vi "determine tempos.vi"(8 "error in (no error)":errorcluster, 11 "midi-file-events in":refnum<class "midi-file-events.lvclass">) -> (0 "error out":errorcluster, 2 "Track data by Track number":T1(c390), 3 "midi-file-events out":refnum<class "midi-file-events.lvclass">)   [LabVIEW 2020, in "midi-file-events.lvclass"]
uses:
  midi-file-events.lvclass
  midi-file-event.midi/midi-file-event.midi.lvclass
  C:/code/LabVIEW-MIDI/lv-src/midi-file-event/midi-file-event.lvclass
  midi-file-events.lvclass/midi-file-events.ctl
  midi-file-event/midi-file-event.lvclass/midi-file-event.ctl
  midi-file-event/Delta Tiime.get.vi
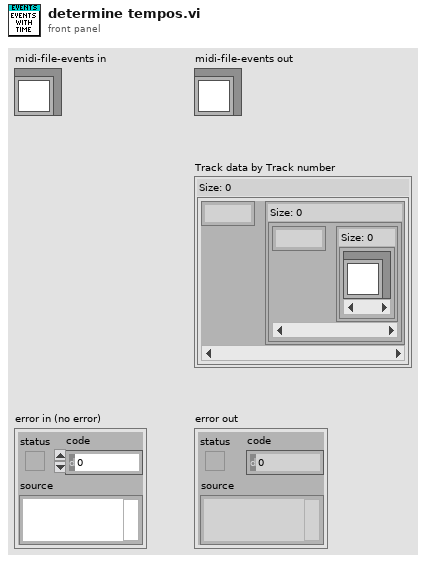
[diagram p1: front panel]
types:
  T1 = map{i32, map{dbl, set{refnum<class "midi-file-event.midi.lvclass">}}}
  T2 = map{dbl, set{refnum<class "midi-file-event.midi.lvclass">}}
  T3 = set{refnum<class "midi-file-event.midi.lvclass">}
  T4 = typedef "midi-file-events.lvclass/privatedata.ctl" = cluster{"ticks per quarter note (division)":i16, "Tempo Map":map{dbl, dbl}, "Track data by Track number":map{i32, map{dbl, set{refnum<class "midi-file-event.midi.lvclass">}}}}
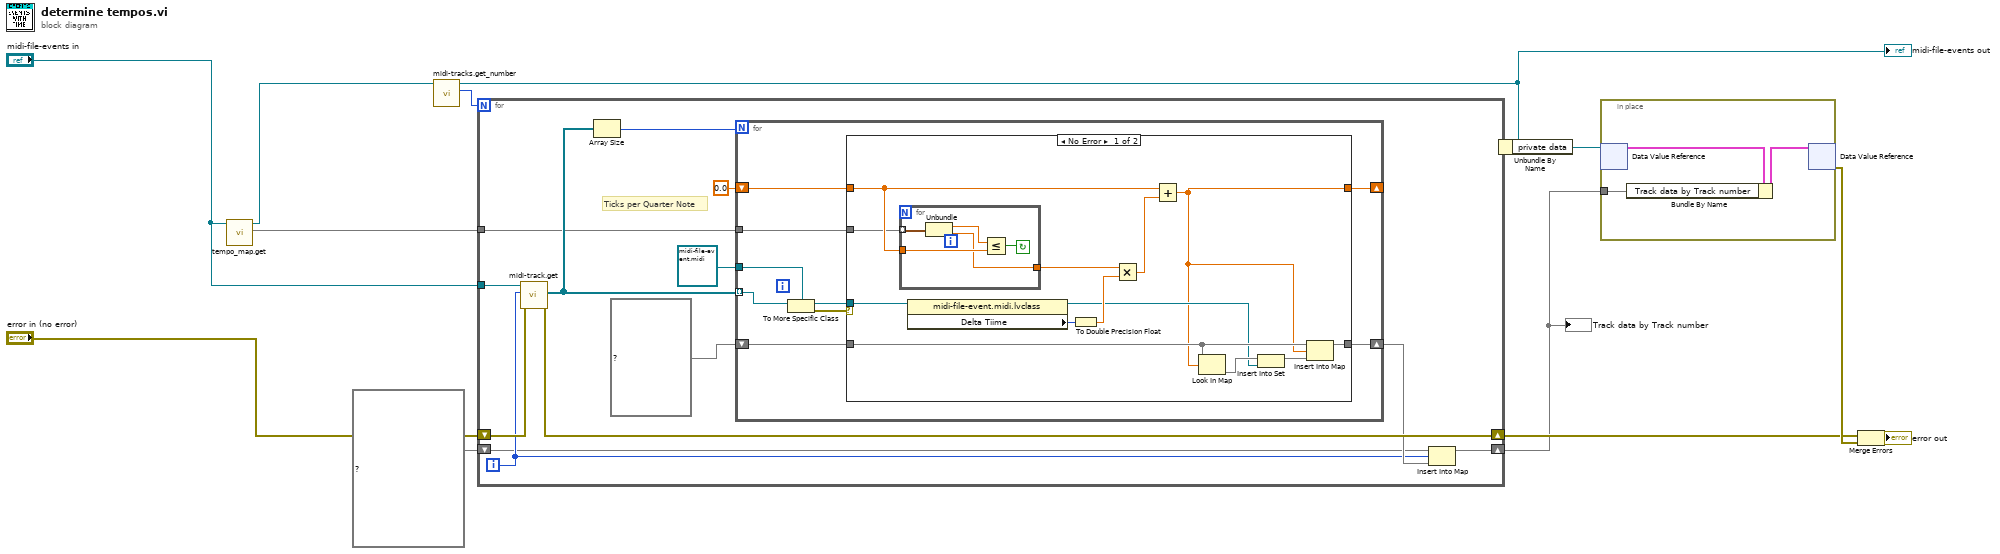
[diagram p0: block diagram]
diagram:
  n1 = call "tempo_map.get.vi"("midi-file-events in"="midi-file-events in") -> ("Tempo Map"=w1:map{dbl, dbl}, "midi-file-events out"=w8:refnum<class "midi-file-events.lvclass">)  [unwired: 8 in, 1 out]
  n2 = call "midi-tracks.get_number.vi"("midi-file-events in"=w8) -> ("Numer of Tracks"=w11:i32, "midi-file-events out"=w7:refnum<class "midi-file-events.lvclass">)  [unwired: 8 in, 1 out]
  "midi-file-events out" <- w7
  n3 = for {
    N: w11 -> [_]
    tunnel: "midi-file-events in" -> [w21]
    shift-right: [w25] -> w4
    shift-left: "error in (no error)" -> [w24]
    shift-right: [w17] -> w2
    shift-left: T1 {} ("Track data by Track number") -> [w18]
    tunnel: w1 -> [w13]
    i -> [w19]
    # "Ticks per Quarter Note"
    n4 = call "midi-track.get.vi"("error in (no error)"=w24, "Track Number"=w19, "midi-file-events in"=w21) -> ("error out"=w25:errorcluster, "file events"=w14:refnum<class "midi-file-event.lvclass">[])  [unwired: 6 in, 1 out]
    n5 = Array Size(array=w14) -> (size(s)=w23:i32)
    n6 = for {
      N: w23 -> [_]
      shift-right: [w33] -> _
      shift-left: 0.0 ("microseconds per quarter note") -> [w34]
      shift-right: [w31] -> w20
      shift-left: T2 {} ("midi event by timestamp") -> [w32]
      tunnel: refnum<class "midi-file-event.midi.lvclass"> refnum ("midi-file-event.midi.lvclass") -> [w30]
      tunnel: w14 -> [w28] mode=indexing
      tunnel: w13 -> [w26]
      n7 = To More Specific Class(target class=w30, reference=w28) -> (specific class reference=w27:refnum<class "midi-file-event.midi.lvclass">, error out=w29:errorcluster)  [unwired: 1 in]
      n8 = case shown="No Error" w29 {
        tunnel: w34 -> [w46 w54]
        tunnel: [w43 w53] -> w31
        tunnel: w32 -> [w42 w53]
        tunnel: [w37 w54] -> w33
        tunnel: w27 -> [w38 _]
        tunnel: w26 -> [w36 _]
        frame No Error {
          n9 = for {
            tunnel: w46 -> [w52]
            tunnel: w36 -> [w50] mode=indexing
            tunnel: [w49] -> w35
            stop <- w51 continue-if-true
            n10 = Unbundle(w50) -> ("Time"=w48:dbl, "Seconds Per Click"=w49:dbl)
            n11 = Less Or Equal?(x=w48, y=w52) -> (x <= y?=w51:bool)
          }
          n12 = property class="midi-file-event.midi.lvclass"(reference=w38) -> (reference out=w40:refnum<class "midi-file-event.midi.lvclass">, "Delta Tiime"=w47:u32)  [unwired: 1 in, 1 out]
          n13 = To Double Precision Float(number=w47) -> (double precision float=w45:dbl)
          n14 = Multiply(x=w35, y=w45) -> (x*y=w44:dbl)
          n15 = Add(x=w46, y=w44) -> (x+y=w37:dbl)
          n16 = Look In Map(map=w42, key=w37) -> (value=w41:T3)  [unwired: 1 in, 1 out]
          n17 = Insert Into Set(10:w40, 11:w41) -> (3:w39:T3)  [unwired: 1 out]
          n18 = Insert Into Map(map in=w42, key=w37, value=w39) -> (map out=w43:T2)  [unwired: 2 out]
        }
        frame Error {
        }
      }
    }
    n19 = Insert Into Map(map in=w18, key=w19, value=w20) -> (map out=w17:T1)  [unwired: 2 out]
  }
  "Track data by Track number" <- w2
  n20 = Unbundle By Name(w7) -> ("private data"=w6:refnum<data-value>)
  n21 = in-place {
    in-place-border: w2 -> [w55]
    n22 = in-place-dvr #1(w6) -> (w57:T4)  [unwired: 1 out]
    n23 = Bundle By Name(cluster=w57, "Track data by Track number"=w55) -> (w56:T4)
    n24 = in-place-dvr #1(w56) -> (w5:errorcluster)  [unwired: 1 out]
  }
  n25 = Merge Errors(w4, w5) -> (→"error out":errorcluster)
